vi "test Convert Endpoint to UI Element.vi"(8 "error in (no error)":errorcluster, 11 "TestCase in":refnum<class "SLSC Switch Unit Tests.lvclass">) -> (0 "error out":errorcluster, 3 "TestCase out":refnum<class "SLSC Switch Unit Tests.lvclass">)   [LabVIEW 2017, in "SLSC Switch Unit Tests.lvclass"]
uses:
  SLSC Switch Unit Tests.lvclass
  Shared/Endpoint Configuration Enum.ctl
  System Explorer/Channel Type.ctl
  Shared/Endpoint Configuration Cluster.ctl
  <vilib>/addons/_JKI Toolkits/VI Tester/TestCase.llb/TestCase.lvclass
  System Explorer/SLSC Switch System Explorer.lvlib
  Shared/SLSC Switch Shared.lvlib
  C:/Program Files (x86)/National Instruments/LabVIEW 2017/vi.lib/addons/_JKI Toolkits/VI Tester/TestCase.llb/TestCase.lvclass
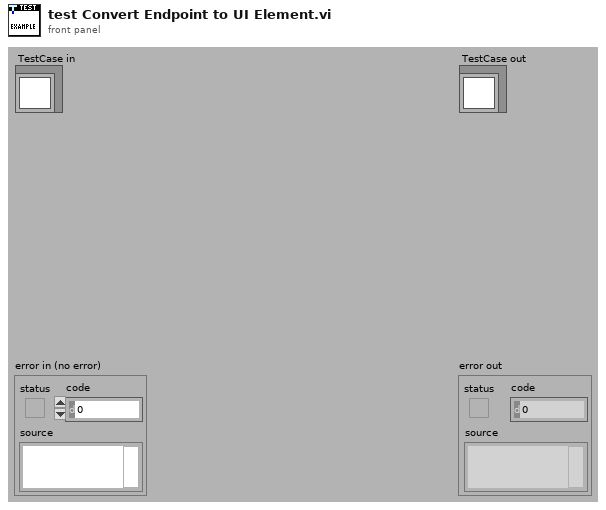
[diagram p1: front panel]
types:
  T1 = typedef "SLSC Switch Shared.lvlib/Endpoint Configuration Enum.ctl" = enum16{"Load", "Source", "Configuration"}
  T2 = typedef "SLSC Switch System Explorer.lvlib/Channel Type.ctl" = enum16{"Load (Default)", "Source", "Configuration"}
  T3 = cluster{"Configuration":T1, "Configuration 2":T2}[]
  T4 = typedef "SLSC Switch Shared.lvlib/Endpoint Configuration Cluster.ctl" = cluster{"Endpoint":string, "Configuration":T1}
  T5 = typedef "SLSC Switch System Explorer.lvlib/Channel.ctl" = cluster{"Endpoint":string, "Configuration":T2}
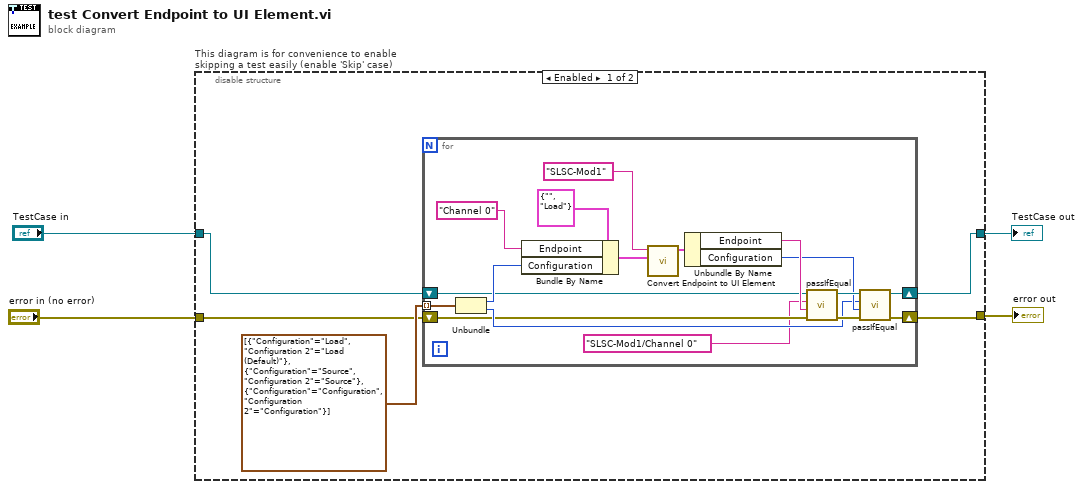
[diagram p0: block diagram]
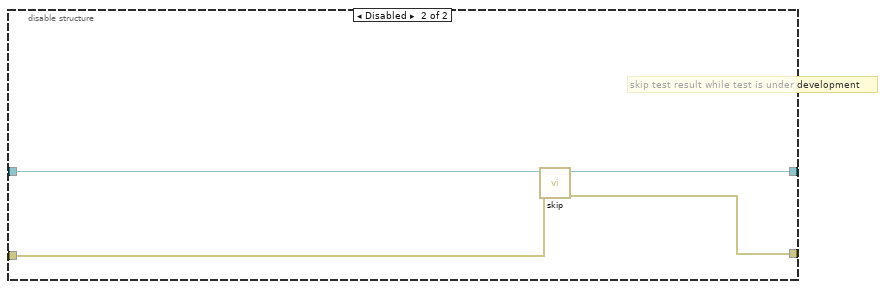
[diagram p2: hidden frame]
diagram:
  n1 = disable-structure "This diagram is for convenience to enable skipping a test easily (enable 'Skip' case)" shown="Enabled" {
    disable-tunnel: "TestCase in" -> [w6 w30]
    disable-tunnel: [w5 w28] -> w1
    disable-tunnel: [w7 w29] -> w3
    disable-tunnel: "error in (no error)" -> [w8 w27]
    frame Enabled {
      n2 = for {
        tunnel: T3 [{"Configuration"=enum."Load", "Configuration 2"=enum."Load (Default)"}, {"Configuration"=enum."Source", "Configuration 2"=enum."Source"}, {"Configuration"=enum."Configuration", "Configuration 2"=enum."Configuration"}] -> [w19] mode=indexing
        shift-right: [w15] -> w7
        shift-left: w8 -> [w16]
        shift-right: [w13] -> w5
        shift-left: w6 -> [w14]
        n3 = Unbundle(w19) -> ("Configuration"=w18:T1, "Configuration 2"=w17:T2)
        n4 = Bundle By Name(cluster=T4 {"Endpoint"="", "Configuration"=enum."Load"} ("Connection"), "Endpoint"="Channel 0", "Configuration"=w18) -> (w11:T4)
        n5 = call "Convert Endpoint to UI Element.vi"("Connection"=w11, "Resource"="SLSC-Mod1") -> ("Channel"=w26:T5)  [unwired: 9 in]
        n6 = Unbundle By Name(w26) -> ("Endpoint"=w22:string, "Configuration"=w20:T2)
        n7 = call-dynamic "passIfEqual.vi"("error in (no error)"=w16, "y"=w22, "x"="SLSC-Mod1/Channel 0" ("Resource"), "TestCase in"=w14) -> ("error out"=w23:errorcluster, "TestCase out"=w24:refnum<class "SLSC Switch Unit Tests.lvclass">)  [unwired: 6 in]
        n8 = call-dynamic "passIfEqual.vi"("error in (no error)"=w23, "y"=w20, "x"=w17, "TestCase in"=w24) -> ("error out"=w15:errorcluster, "TestCase out"=w13:refnum<class "SLSC Switch Unit Tests.lvclass">)  [unwired: 6 in]
      }
    }
    frame Disabled {
      # "skip test result while test is under development"
      n9 = call <vilib>:"skip.vi"("error in (no error)"=w27, "TestCase in"=w30) -> ("error out"=w29:errorcluster, "TestCase out"=w28:refnum<class "SLSC Switch Unit Tests.lvclass">)  [unwired: 8 in]
    }
  }
  "error out" <- w3
  "TestCase out" <- w1
